vi "initialize.vi"(8 "error in":errorcluster, 11 "configuration in":refnum<class "NISE_CEF_serializable configuration.lvclass">) -> (0 "error out":errorcluster, 2 "identifier":string, 3 "configuration out":refnum<class "NISE_CEF_serializable configuration.lvclass">)   [LabVIEW 2013, in "NISE_CEF_serializable configuration.lvclass"]
uses:
  NISE_CEF_serializable configuration.lvclass
  NISE_CEF_serializable configuration.lvclass/NISE_CEF_serializable configuration.ctl
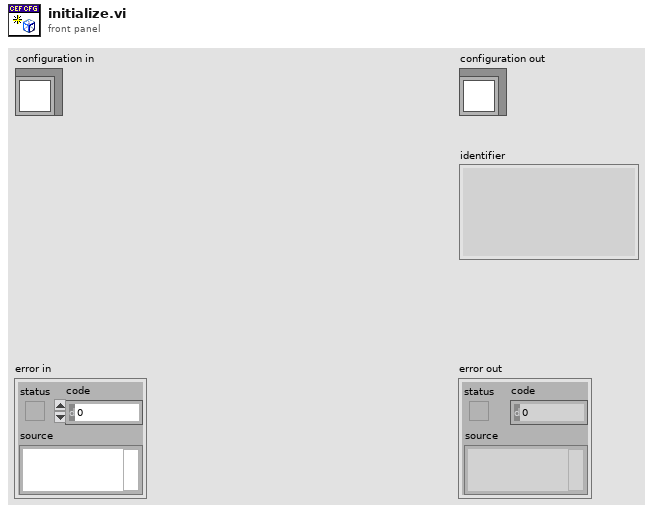
[diagram p1: front panel]
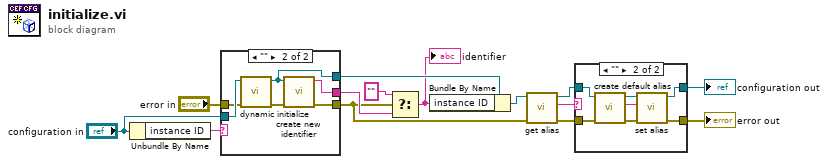
[diagram p0: block diagram]
diagram:
  n1 = Unbundle By Name("configuration in") -> ("instance ID"=w14:string)
  n2 = case shown="\"\"" w14 {
    selector: w14 -> [w17 _]
    tunnel: [w17 w23] -> w10
    tunnel: "configuration in" -> [w16 w22]
    tunnel: "error in" -> [w15 w21]
    tunnel: [w15 w19] -> w6
    tunnel: [w16 w18] -> w11
    frame Default {
    }
    frame "" {
      n3 = call-dynamic "dynamic initialize.vi"("error in"=w21, "configuration in"=w22) -> ("error out"=w20:errorcluster, "configuration out"=w18:refnum<class "NISE_CEF_serializable configuration.lvclass">)  [unwired: 8 in]
      n4 = call-dynamic "create new identifier.vi"("error in"=w20, "configuration in"=w18) -> ("error out"=w19:errorcluster, "id"=w23:string)  [unwired: 8 in]
    }
  }
  n5 = Select(t="", s=w6, f=w10) -> (s? t:f=w8:string)
  "identifier" <- w8
  n6 = Bundle By Name(cluster=w11, "instance ID"=w8) -> (w7:refnum<class "NISE_CEF_serializable configuration.lvclass">)
  n7 = call "get alias.vi"("error in"=w6, "configuration in"=w7) -> ("error out"=w4:errorcluster, "alias"=w5:string, "configuration out"=w1:refnum<class "NISE_CEF_serializable configuration.lvclass">)  [unwired: 7 in]
  n8 = case shown="\"\"" w5 {
    tunnel: w4 -> [w24 w30]
    tunnel: [w24 w28] -> w3
    tunnel: [w25 w27] -> w2
    tunnel: w1 -> [w25 w26]
    frame Default {
    }
    frame "" {
      n9 = call-dynamic "create default alias.vi"("error in"=w30, "configuration in"=w26) -> ("error out"=w31:errorcluster, "default alias"=w29:string, "configuration out"=w32:refnum<class "NISE_CEF_serializable configuration.lvclass">)  [unwired: 7 in]
      n10 = call "set alias.vi"("error in"=w31, "alias"=w29, "configuration in"=w32) -> ("error out"=w28:errorcluster, "configuration out"=w27:refnum<class "NISE_CEF_serializable configuration.lvclass">)  [unwired: 7 in]
    }
  }
  "error out" <- w3
  "configuration out" <- w2
